vi "Write Active Cell Cell Justification.vi"(8 "error in (no error)":errorcluster, 10 "CellJustify":enum16{"Left", "Center", "Right"}(ring), 11 "Table.lvclass in":refnum<class "Table.lvclass">) -> (0 "error out":errorcluster, 3 "Table.lvclass out":refnum<class "Table.lvclass">)   [LabVIEW 2015, in "Table.lvclass"]
uses:
  Table.lvclass
  Table.lvclass/Table.ctl
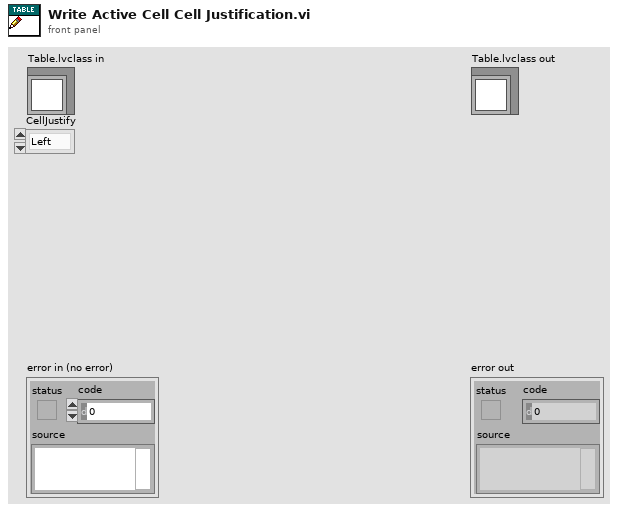
[diagram p1: front panel]
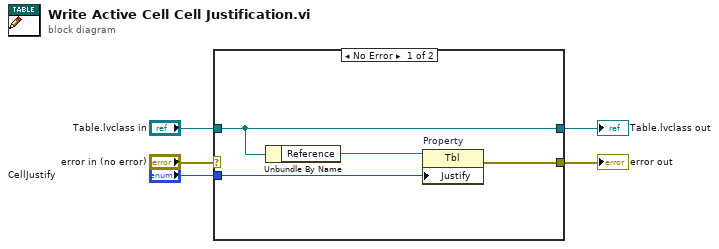
[diagram p0: block diagram]
diagram:
  n1 = case shown="No Error" "error in (no error)" {
    selector: "error in (no error)" -> [_ w11]
    tunnel: [w9 w11] -> w4
    tunnel: [w7 w10] -> w2
    tunnel: "Table.lvclass in" -> [w7 w10]
    tunnel: "CellJustify" -> [w8 _]
    frame No Error {
      n2 = Unbundle By Name(w7) -> ("Reference"=w6:refnum<vi>)
      n3 = property on="Property" class="Tbl"(reference=w6, "Justify"=w8) -> (error out=w9:errorcluster)  [unwired: 1 in, 1 out]
    }
    frame Error {
    }
  }
  "error out" <- w4
  "Table.lvclass out" <- w2
